vi "Calculadora.vi"() -> ()   [LabVIEW 2019]
panel:
  out "Alerta":string
  out "Resultado":dbl
  in  "Division":bool
  in  "Resta":bool
  in  "Multiplicacion":bool
  in  "Suma":bool
  in  "Numero 2":dbl
  in  "Numero 1":dbl
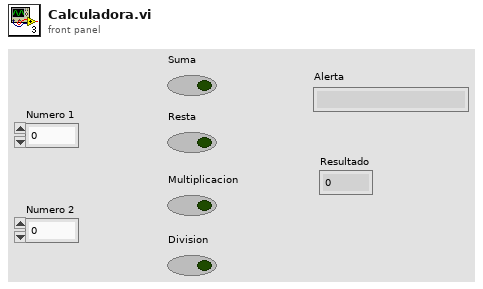
[diagram p1: front panel]
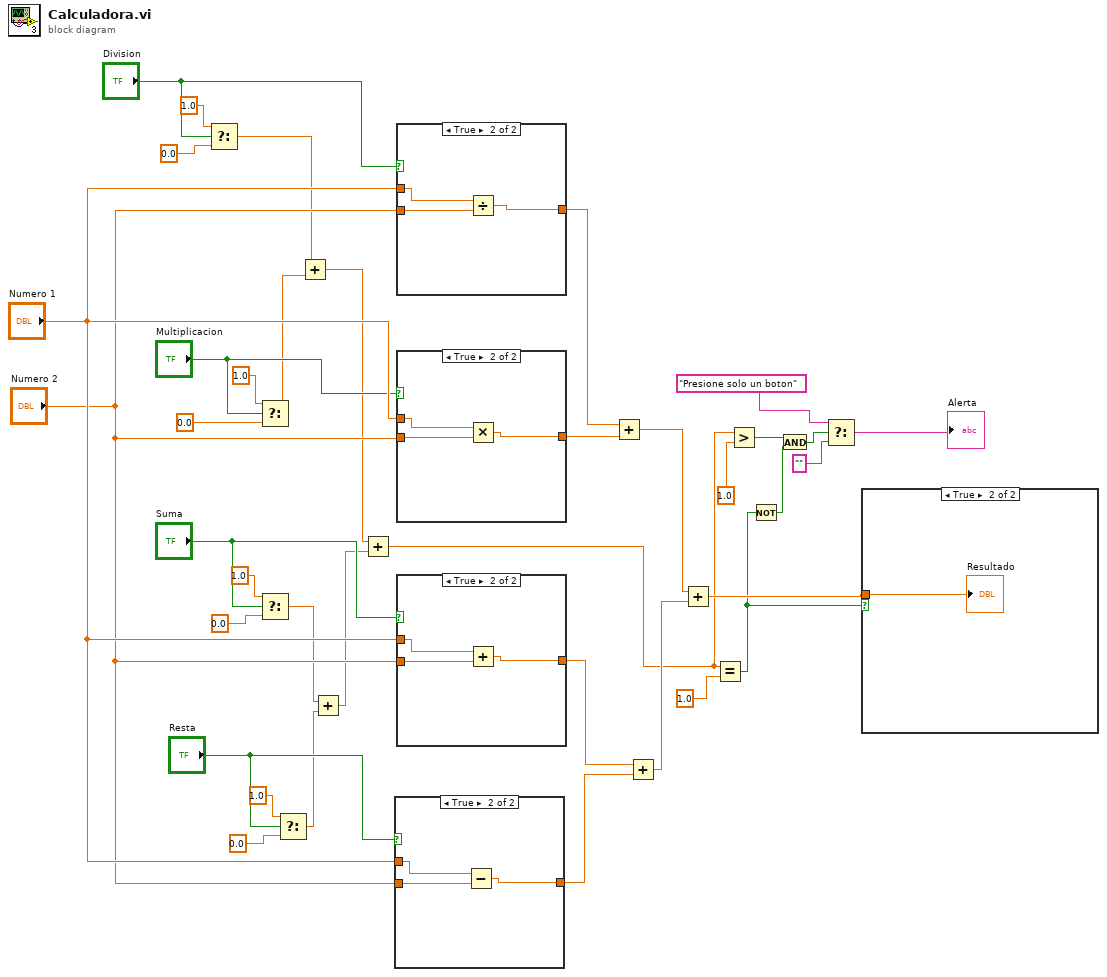
[diagram p0: block diagram]
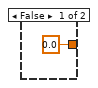
[diagram p3: hidden frame]
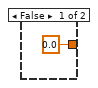
[diagram p4: hidden frame]
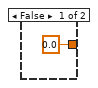
[diagram p5: hidden frame]
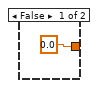
[diagram p6: hidden frame]
diagram:
  n1 = Select(t=1.0, s="Division", f=0.0) -> (s? t:f=w27:dbl)
  n2 = Select(t=1.0, s="Multiplicacion", f=0.0) -> (s? t:f=w23:dbl)
  n3 = Select(t=1.0, s="Suma", f=0.0) -> (s? t:f=w15:dbl)
  n4 = Select(t=1.0, s="Resta", f=0.0) -> (s? t:f=w16:dbl)
  n5 = Add(x=w27, y=w23) -> (x+y=w13:dbl)
  n6 = Add(x=w15, y=w16) -> (x+y=w14:dbl)
  n7 = Add(x=w13, y=w14) -> (x+y=w4:dbl)
  n8 = case shown="True" "Resta" {
    tunnel: "Numero 1" -> [_ w41]
    tunnel: "Numero 2" -> [_ w40]
    tunnel: [0.0 w39] -> w32
    frame False {
    }
    frame True {
      n9 = Subtract(x=w41, y=w40) -> (x-y=w39:dbl)
    }
  }
  n10 = case shown="True" "Division" {
    tunnel: "Numero 1" -> [_ w45]
    tunnel: "Numero 2" -> [_ w44]
    tunnel: [0.0 w43] -> w36
    frame False {
    }
    frame True {
      n11 = Divide(x=w45, y=w44) -> (x/y=w43:dbl)
    }
  }
  n12 = case shown="True" "Multiplicacion" {
    tunnel: "Numero 1" -> [_ w49]
    tunnel: "Numero 2" -> [_ w48]
    tunnel: [0.0 w47] -> w37
    frame False {
    }
    frame True {
      n13 = Multiply(x=w49, y=w48) -> (x*y=w47:dbl)
    }
  }
  n14 = case shown="True" "Suma" {
    tunnel: "Numero 1" -> [_ w53]
    tunnel: "Numero 2" -> [_ w52]
    tunnel: [0.0 w51] -> w33
    frame False {
    }
    frame True {
      n15 = Add(x=w53, y=w52) -> (x+y=w51:dbl)
    }
  }
  n16 = Add(x=w36, y=w37) -> (x+y=w10:dbl)
  n17 = Add(x=w33, y=w32) -> (x+y=w31:dbl)
  n18 = Add(x=w10, y=w31) -> (x+y=w11:dbl)
  n19 = Equal?(x=w4, y=1.0) -> (x = y?=w9:bool)
  n20 = Greater?(x=w4, y=1.0) -> (0:w5:bool)
  n21 = Not(x=w9) -> (.not. x?=w2:bool)
  n22 = And(x=w5, y=w2) -> (x .and. y?=w1:bool)
  n23 = Select(t="Presione solo un boton", s=w1, f="") -> (s? t:f=→"Alerta":string)
  n24 = case shown="True" w9 {
    tunnel: w11 -> [_ w54]
    frame False {
    }
    frame True {
      "Resultado" <- w54
    }
  }
